vi "rwfm_BufferCfg.vi"(8 "error in":errorcluster, 9 "Buffer Size [Samps per Chan]":i32=500000, 10 "Sampling Info In":T2, 11 "Dynamic FPGA VI Reference":T1) -> (0 "error out":errorcluster, 1 "Buffer Size [Total Samples]":u32=500000, 2 "Sampling Info Out":T2, 3 "Dynamic FPGA VI Reference":T1)   [LabVIEW 2017, in "cRIOWfmLibMcsa.lvlib"]
doc: "This VI sets the host application's data buffer size, which is critical for maximum data throughput. This buffer is responsible for receiving data coming from the FPGA DMA FIFO. For the continuous case the buffer size should be many times larger than your read size. In the finite case, the timing VIs automatically call this VI and set the buffer size equal to the number of samples in the acquisition."
uses:
  <vilib>/addons/InsightCM/Devices/Shared/Mcsa/cRIOWfmAcqMcsa/cRIOWfmLibMcsa.lvlib
  <vilib>/addons/InsightCM/Devices/Shared/Cms/cRIOWfmAcq/subVIs/RIO Wfm Cust Ctrls/rwfm_SamplingInfo.ctl
  <vilib>/addons/InsightCM/Devices/Shared/Mcsa/cRIOWfmAcqMcsa/controls/rwfm_DynamicFPGArefMCSA.ctl
  <vilib>/rvi/interface/common/niFpgaWaitOnOcc.vi
  <vilib>/Utility/error.llb/Error Cluster From Error Code.vi
  <vilib>/rvi/interface/nirviMethod/nirviMethod.xnode
  <vilib>/rvi/errors/niLvFpgaMergeErrorWithErrorCode.vi
  <vilib>/FPGAPlugInAG/Dynamic/niLvFpga_ConfigureFifo_Dynamic.vi
  <vilib>/FPGAPlugInAG/Dynamic/niLvFpga_StartFifo_Dynamic.vi
  <vilib>/addons/InsightCM/Devices/Shared/Cms/cRIOWfmAcq/cRIOWfmLib.lvlib
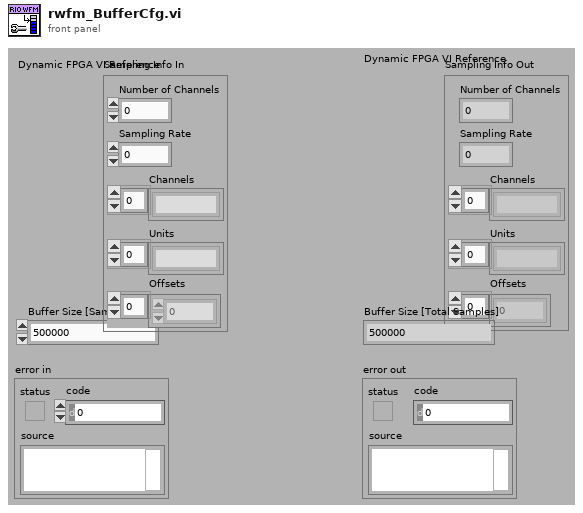
[diagram p1: front panel]
types:
  T1 = typedef "cRIOWfmLibMcsa.lvlib/rwfm_DynamicFPGArefMCSA.ctl" = refnum<k20>
  T2 = typedef "cRIOWfmLib.lvlib/rwfm_SamplingInfo.ctl" = cluster{"Number of Channels":i32, "Sampling Rate":dbl, "Channels":string[], "Units":string[], "Offsets":sgl[]}
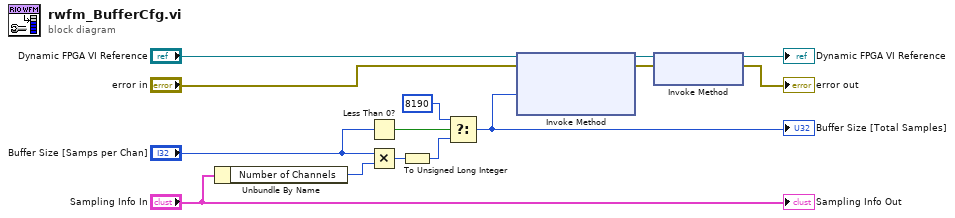
[diagram p0: block diagram]
diagram:
  n1 = Unbundle By Name("Sampling Info In") -> ("Number of Channels"=w12:i32)
  n2 = Less Than 0?(x="Buffer Size [Samps per Chan]") -> (x < 0?=w7:bool)
  n3 = Multiply(x="Buffer Size [Samps per Chan]", y=w12) -> (x*y=w11:i32)
  n4 = To Unsigned Long Integer(number=w11) -> (unsigned 32bit integer=w10:u32)
  n5 = Select(t=u32 8190 ("unsigned 32bit integer"), s=w7, f=w10) -> (s? t:f=w1:u32)
  "Buffer Size [Total Samples]" <- w1
  n6 = xnode "Invoke Method"("FPGA VI Reference In"="Dynamic FPGA VI Reference", "error in"="error in", "Requested Depth"=w1) -> ("FPGA VI Reference Out"=w4:T1, "error out"=w2:errorcluster)  [unwired: 1 out]
  n7 = xnode "Invoke Method"("FPGA VI Reference In"=w4, "error in"=w2) -> ("FPGA VI Reference Out"=→"Dynamic FPGA VI Reference":T1, "error out"=→"error out":errorcluster)
  "Sampling Info Out" <- "Sampling Info In"
